vi "Get_Box.vi"(7 "Dark Blue \nFrame":T2={"Rmax"=14.0, "Rmin"=0.0, "Gmax"=42.0, "Gmin"=0.0, "Bmax"=126.0, "Bmin"=121.0}, 8 "Error in (no error)":errorcluster, 11 "Path to PNG file":path) -> (0 "Error out":errorcluster, 2 "BillardBox":T1)   [LabVIEW 2019]
doc: "Get_Box.vi\nFind the coordinates of billard box by iteration with two nested loop.\nInput : -Path to PNG file\n -Dark Blue Frame containing the range of colors of the edge \n -Error in\nOutput : -BillardBox containing the coordinates of the billard box\n -Error out"
panel:
  in  "Initial BillardBox":T1
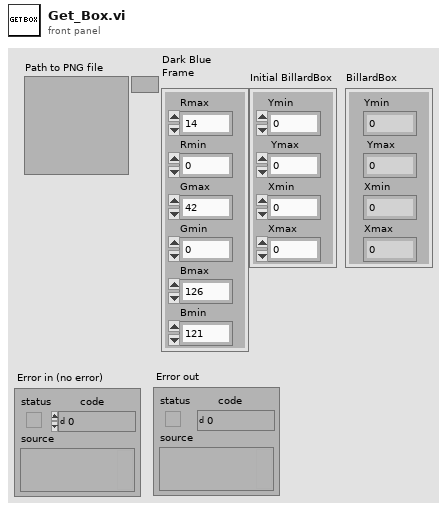
[diagram p1: front panel]
types:
  T1 = cluster{"Ymin":dbl, " Ymax":dbl, "Xmin":dbl, "Xmax":dbl}
  T2 = cluster{"Rmax":dbl, "Rmin":dbl, "Gmax":dbl, "Gmin":dbl, "Bmax":dbl, "Bmin":dbl}
  T3 = typedef "imagedata.ctl" = cluster{"image type":i32, "image depth":i32, "image":u8[], "mask":u8[], "colors":u32[], "Rectangle":cluster{"left":i16, "top":i16, "right":i16, "bottom":i16}}
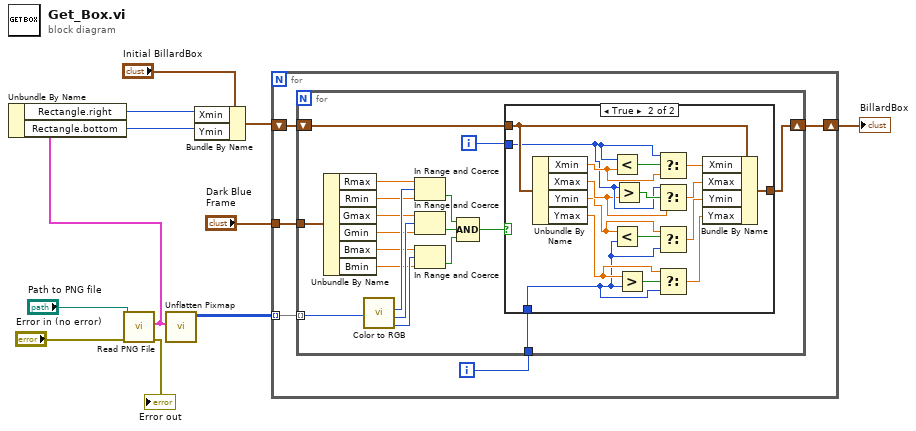
[diagram p0: block diagram]
diagram:
  n1 = call <vilib>:"Read PNG File.vi"("error in (no error)"="Error in (no error)", "path to PNG file"="Path to PNG file") -> ("error out"=→"Error out":errorcluster, "image data"=w8:T3)  [unwired: 7 in, 1 out]
  n2 = Unbundle By Name(w8) -> ("Rectangle.right"=w7:i16, "Rectangle.bottom"=w6:i16)
  n3 = call <vilib>:"Unflatten Pixmap.vi"("image data"=w8) -> ("24-bit pixmap"=w11:u32[][])  [unwired: 4 in, 6 out]
  n4 = Bundle By Name(cluster="Initial BillardBox", "Xmin"=w7, "Ymin"=w6) -> (w9:T1)
  n5 = for {
    tunnel: w11 -> [w16] mode=indexing
    tunnel: "Dark Blue \nFrame" -> [w15]
    shift-right: [w14] -> w1
    shift-left: w9 -> [w12]
    i -> [w13]
    n6 = for {
      tunnel: w16 -> [w29] mode=indexing
      tunnel: w15 -> [w26]
      shift-right: [w18] -> w14
      shift-left: w12 -> [w27]
      tunnel: w13 -> [w17]
      i -> [w28]
      n7 = Unbundle By Name(w26) -> ("Rmax"=w25:dbl, "Rmin"=w24:dbl, "Gmax"=w23:dbl, "Gmin"=w22:dbl, "Bmax"=w21:dbl, "Bmin"=w20:dbl)
      n8 = call <vilib>:"Color to RGB.vi"("Color"=w29) -> ("R"=w35:u8, "G"=w34:u8, "B"=w33:u8)  [unwired: 1 out]
      n9 = In Range and Coerce(upper limit=w25, x=w35, lower limit=w24) -> (In Range?=w32:bool)  [unwired: 1 out]
      n10 = In Range and Coerce(upper limit=w23, x=w34, lower limit=w22) -> (In Range?=w31:bool)  [unwired: 1 out]
      n11 = In Range and Coerce(upper limit=w21, x=w33, lower limit=w20) -> (In Range?=w30:bool)  [unwired: 1 out]
      n12 = Compound Arithmetic op=AND(w32, w31, w30) -> (w19:bool)
      n13 = case shown="True" w19 {
        tunnel: w28 -> [_ w43]
        tunnel: w27 -> [w36 w52]
        tunnel: [w36 w51] -> w18
        tunnel: w17 -> [_ w37]
        frame False {
        }
        frame True {
          n14 = Unbundle By Name(w52) -> ("Xmin"=w45:dbl, "Xmax"=w42:dbl, "Ymin"=w39:dbl, "Ymax"=w41:dbl)
          n15 = Less?(x=w43, y=w45) -> (x < y?=w46:bool)
          n16 = Less?(x=w39, y=w37) -> (x < y?=w38:bool)
          n17 = Greater?(x=w43, y=w42) -> (0:w44:bool)
          n18 = Greater?(x=w41, y=w37) -> (0:w40:bool)
          n19 = Select(t=w43, s=w46, f=w45) -> (s? t:f=w50:dbl)
          n20 = Select(t=w43, s=w44, f=w42) -> (s? t:f=w49:dbl)
          n21 = Select(t=w39, s=w38, f=w37) -> (s? t:f=w48:dbl)
          n22 = Select(t=w41, s=w40, f=w37) -> (s? t:f=w47:dbl)
          n23 = Bundle By Name(cluster=w52, "Xmin"=w50, "Xmax"=w49, "Ymin"=w48, "Ymax"=w47) -> (w51:T1)
        }
      }
    }
  }
  "BillardBox" <- w1
